vi "Zmienna Temp FGV.vi"(7 "Akcje (GET)":T1=enum."GET", 8 "error in (no error)":errorcluster, 9 "Temp limits in":T2={"Max (25)"=25.0, "Min (0)"=0.0}, 11 "Zakres in":i32=5) -> (0 "error out":errorcluster, 1 "Temp limits out":T2={"Max (25)"=25.0, "Min (0)"=0.0}, 3 "Zakres out":i32=5)   [LabVIEW 2013]
doc: "Przenosi zmienne z pêtli GUI do Przetwrzanie"
uses:
  inne pliki/Params.ctl
  inne pliki/Akcje rownolegle FVG.ctl
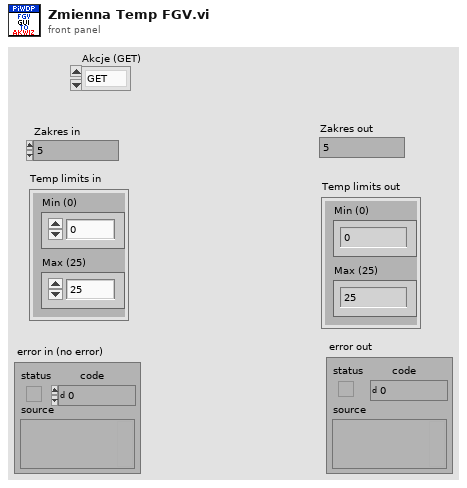
[diagram p1: front panel]
types:
  T1 = typedef "Akcje rownolegle FVG.ctl" = enum16{"SET", "GET"}
  T2 = typedef "Params.ctl" = cluster{"Max (25)":dbl, "Min (0)":dbl}
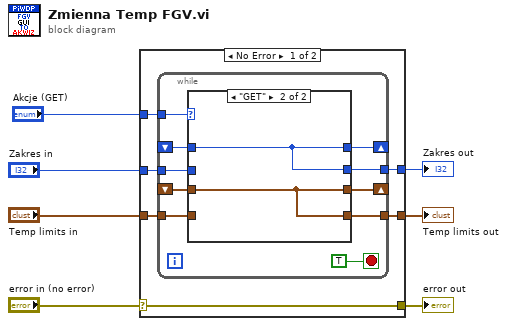
[diagram p0: block diagram]
diagram:
  n1 = case shown="No Error" "error in (no error)" {
    selector: "error in (no error)" -> [w13 w30]
    tunnel: [w13 w30] -> w6
    tunnel: "Zakres in" -> [w12 w29]
    tunnel: "Temp limits in" -> [w11 w28]
    tunnel: [w10 w28] -> w3
    tunnel: [w9 w29] -> w2
    tunnel: "Akcje (GET)" -> [w8 _]
    frame No Error {
      n2 = while {
        tunnel: w12 -> [w23]
        tunnel: w11 -> [w22]
        shift-right: [w20] -> _
        shift-left: _ -> [w15]
        shift-right: [w19] -> _
        shift-left: _ -> [w14]
        tunnel: [w18] -> w10
        tunnel: [w17] -> w9
        tunnel: w8 -> [w16]
        stop <- TRUE stop-if-true
        n3 = case shown="\"GET\"" w16 {
          tunnel: w23 -> [w24 _]
          tunnel: w22 -> [w25 _]
          tunnel: [w24 w27] -> w20
          tunnel: [w25 w26] -> w19
          tunnel: [w25 w26] -> w18
          tunnel: [w24 w27] -> w17
          tunnel: w15 -> [_ w27]
          tunnel: w14 -> [_ w26]
          frame "SET", Default {
          }
          frame "GET" {
          }
        }
      }
    }
    frame Error {
    }
  }
  "error out" <- w6
  "Zakres out" <- w2
  "Temp limits out" <- w3
